vi "Begin.vi"(11 "Image Size":T1=enum."160x120") -> (0 "error out":errorcluster)   [LabVIEW 2013]
doc: "Called before other user functions, this VI is expected to open initial I/O refnums, load in file data, and do all program initialization. Notice that the <B>error out</B> terminal is simply used for data flow. Wiring it to other structures or subVIs ensures that this VI runs first."
uses:
  <vilib>/Rock Robotics/WPI/Camera/WPI_CameraImageSize.ctl
  <vilib>/Rock Robotics/WPI/Camera/WPI_CameraWhite Balance Values.ctl
  <vilib>/Rock Robotics/WPI/Camera/WPI_CameraExposure Values.ctl
  <vilib>/Rock Robotics/WPI/Camera/WPI_CameraFrameRate.ctl
  <vilib>/Rock Robotics/WPI/DriverStation/WPI_DriverStationRobotMode2.ctl
  <vilib>/Rock Robotics/SystemInterfaces/DIO/FPGA_DIOPWMChannel.ctl
  <vilib>/Rock Robotics/WPI/SafetyOutput/WPI_SafetyOutputConfigMenu.ctl
  <vilib>/Rock Robotics/WPI/Joystick/WPI_JoystickDeviceEnum.ctl
  TankDriveEnum.ctl
  Robot Global Data.vi
  <vilib>/Rock Robotics/WPI/RobotDrive/WPI_RobotDriveOpen2MotorWithTalon.vi
  <vilib>/Rock Robotics/WPI/Counter/WPI_CounterDigitalInputToDigitalSource.vi
  <vilib>/Rock Robotics/SystemInterfaces/Typedef/FPGA_TypedefDigitalModule.ctl
  <vilib>/Rock Robotics/SystemInterfaces/DIO/FPGA_DIOChannel.ctl
  <vilib>/Rock Robotics/WPI/Encoder/WPI_EncoderType.ctl
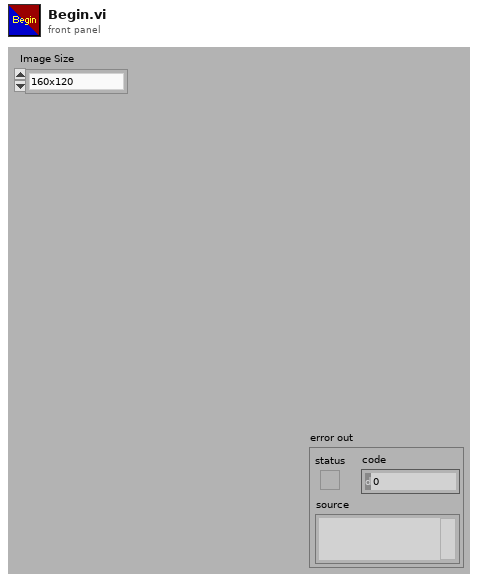
[diagram p1: front panel]
types:
  T1 = typedef "WPI_CameraImageSize.ctl" = enum16{"640x480", "320x240", "160x120"}
  T2 = typedef "TankDriveEnum.ctl" = enum16{"Init", "SetValue", "Disable", "Linear Drive"}
  T3 = typedef "WPI_JoystickDeviceEnum.ctl" = enum16{"USB 1", "USB 2", "USB 3", "USB 4", "Kinect 1", "Kinect 2"}
  T4 = typedef "WPI_SafetyOutputConfigMenu.ctl" = enum16{"Enable", "Disable"}
  T5 = typedef "FPGA_DIOPWMChannel.ctl" = enum8{"PWM 1", "PWM 2", "PWM 3", "PWM 4", "PWM 5", "PWM 6", "PWM 7", "PWM 8", "PWM 9", "PWM 10", "Invalid"}
  T6 = typedef "WPI_DriverStationRobotMode2.ctl" = enum16{"Autonomous Disabled", "Autonomous Enabled", "Teleop Disabled", "Teleop Enabled", "Timeout", "Finish", "Test Disabled", "Test Enabled"}
  T7 = typedef "WPI_CameraFrameRate.ctl" = u32
  T8 = typedef "WPI_CameraExposure Values.ctl" = enum16{"Auto", "Flicker-free 50 Hz", "Flicker-free 60 Hz", "Hold current"}
  T9 = typedef "WPI_CameraWhite Balance Values.ctl" = enum16{"Auto", "Fixed indoor", "Fixed outdoor 1", "Fixed outdoor 2", "Fixed fluorescent 1", "Fixed fluorescent 2", "Hold current"}
  T10 = typedef "WPI_CameraDevRef.ctl" = cluster{"Camera Address":string, "CameraStatus":errorcluster, "Acquire Image Notifier":refnum<notifier>}
  T11 = typedef "WPI_JoystickDevRef.ctl" = cluster{"Device":T3}
  T12 = typedef "FPGA_DIOChannel.ctl" = enum8{"DIO 1", "DIO 2", "DIO 3", "DIO 4", "DIO 5", "DIO 6", "DIO 7", "DIO 8", "DIO 9", "DIO 10", "DIO 11", "DIO 12", "DIO 13", "DIO 14", "Invalid"}
  T13 = typedef "FPGA_TypedefDigitalModule.ctl" = enum16{"Digital Module 1", "Digital Module 2"}
  T14 = typedef "WPI_EncoderType.ctl" = enum16{"1x", "2x", "4x"}
  T15 = typedef "WPI_DigitalInputDevRef.ctl" = cluster{"DevStatus":errorcluster, "DIO Channel":T12, "Digital Module":T13}
  T16 = typedef "FPGA_CounterEncoderSourceConvertionLVSourceType.ctl" = cluster{"DevStatus":errorcluster, "AnalogTriggerMode?":bool, "DigitalMode":cluster{"Digital Module":T13, "DIO Channel":T17}, "AnalogTriggerMode":cluster{"AnalogTriggerIndex":T18, "OutputType":T19}}
  T17 = typedef "FPGA_DIODigitalSourceChannel.ctl" = enum8{"DIO 1", "DIO 2", "DIO 3", "DIO 4", "DIO 5", "DIO 6", "DIO 7", "DIO 8", "DIO 9", "DIO 10", "DIO 11", "DIO 12", "DIO 13", "DIO 14", "Disabled"}
  T18 = typedef "FPGA_AnalogTriggerIndex.ctl" = enum8{"Trig 0", "Trig 1", "Trig 2", "Trig 3", "Trig 4", "Trig 5", "Trig 6", "Trig 7", "Invalid"}
  T19 = typedef "FPGA_AnalogTriggerOutType.ctl" = enum16{"InWindow", "TriggerState", "Rising", "Falling"}
  T20 = typedef "WPI_EncoderDevRef.ctl" = cluster{"DevStatus":errorcluster, "EncoderIndex":T21, "CounterIndex":T22, "DistancePerCount":dbl, "Decoding Type":T14}
  T21 = typedef "FPGA_EncoderIdx.ctl" = enum8{"Enc 0", "Enc 1", "Enc 2", "Enc 3", "Invalid"}
  T22 = typedef "FPGA_CounterCtrSystemIndex.ctl" = enum8{"Ctr 0", "Ctr 1", "Ctr 2", "Ctr 3", "Ctr 4", "Ctr 5", "Ctr 6", "Ctr 7", "Invalid"}
  T23 = typedef "WPI_RobotDriveDevRef.ctl" = cluster{"DevStatus":errorcluster, "Motors[]":T24[], "Square Inputs":bool, "Max Output":dbl, "Isochronous":bool}
  T24 = typedef "WPI_MotorControlDeviceRef.ctl" = cluster{"DeviceStatus":errorcluster, "Type":enum16{"PWM", "CAN"}, "PWM":cluster{"Digital Module":T13, "PWM Channel":T5, "DeadBand":T25}, "CAN":cluster{"Device Number":u8, "Control Mode":T26, "Semaphore":T27, "Max Vout":dbl}, "Invert":bool, "TransformRef":T28, "InvTransformRef":T28}
  T25 = typedef "WPI_PWMDeadband.ctl" = cluster{"Name":string, "maxPositivePwm":i32, "minPositivePwm":i32, "centerPwm":i32, "maxNegativePwm":i32, "minNegativePwm":i32, "angularRange":u16}
  T26 = typedef "WPI_CANJaguar_ControlMode.ctl" = enum8{"Percent VBus", "Current", "Speed", "Position", "Voltage"}
  T27 = typedef "Semaphore RefNum" = refnum<k1>
  T28 = typedef "WPI_PWMTransform_ConPane.ctl" = refnum<vi>
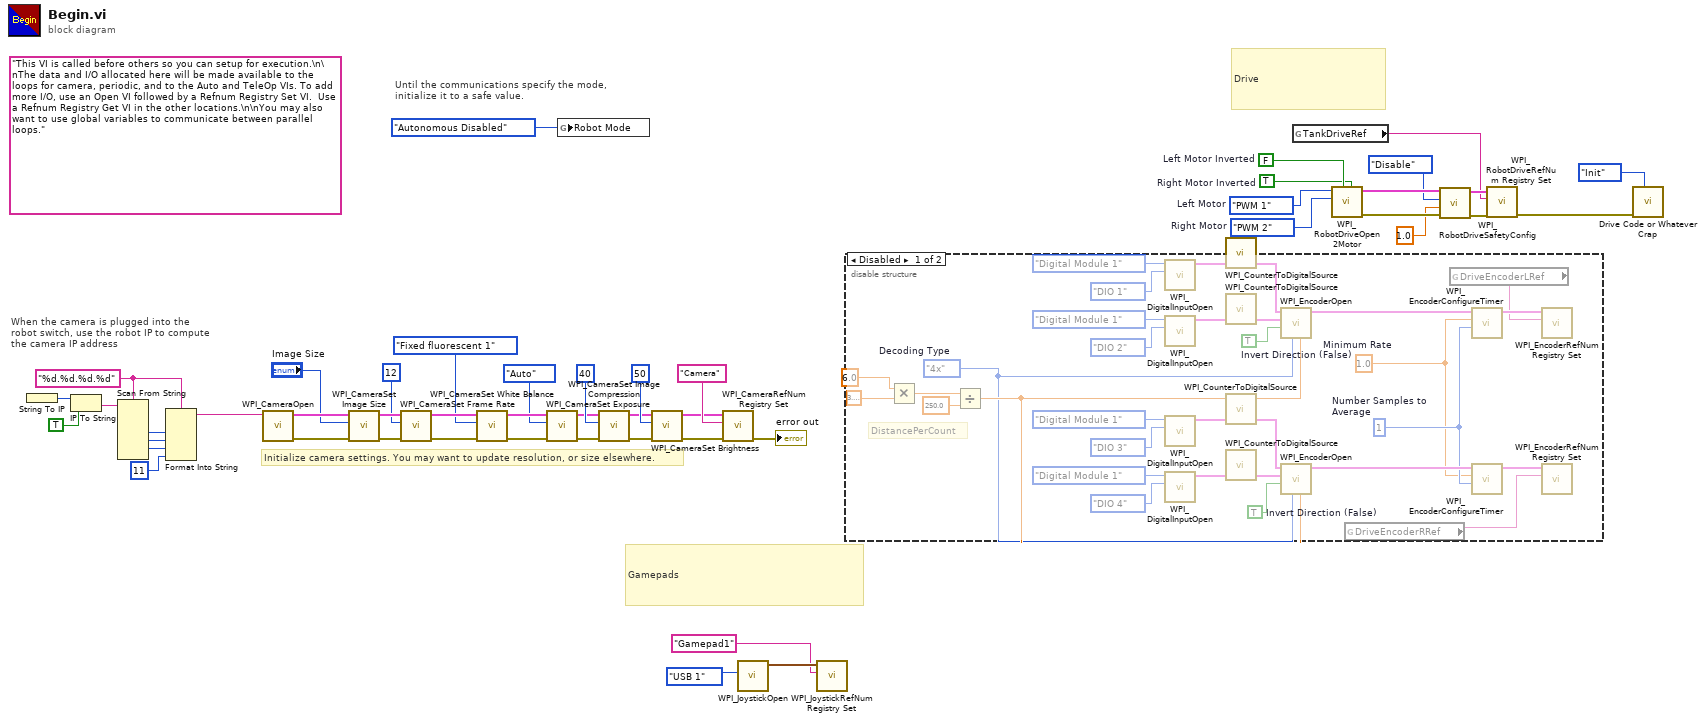
[diagram p0: block diagram]
diagram:
  w13 = FPGA_DIOPWMChannel."PWM 2"  # Right Motor
  w14 = FPGA_DIOPWMChannel."PWM 1"  # Left Motor
  w15 = TRUE  # Right Motor Inverted
  w16 = FALSE  # Left Motor Inverted
  w20 = "%d.%d.%d.%d" ("format string")
  (unwired) "This VI is called before others so you can setup for execution.\n\nThe data and I/O allocated here will be made available to the loops for camera, periodic, and to the Auto and TeleOp VIs. To add more I/O, use an Open VI followed by a Refnum Registry Set VI.  Use a Refnum Registry Get VI in the other locations.\n\nYou may also want to use global variables to communicate between parallel loops."
  # "Gamepads"
  # "Drive"
  # "Until the communications specify the mode,\ninitialize it to a safe value."
  # "When the camera is plugged into the\nrobot switch, use the robot IP to compute\nthe camera IP address"
  # "Initialize camera settings. You may want to update resolution, or size elsewhere."
  n1 = String To IP() -> (0:w27:u32)  [unwired: 1 in]
  n2 = IP To String(1:TRUE ("dot notation? (F)"), 2:w27) -> (0:w25:string)
  n3 = Scan From String(format string=w20, input string=w25) -> (output 1=w24:i32, output 2=w23:i32, output 3=w22:i32)  [unwired: 7 in, 3 out]
  n4 = Format Into String(format string=w20, w24, w23, w22, 11 ("Compression")) -> (resulting string=w18:string)  [unwired: 2 in, 1 out]
  n5 = call <vilib>:"WPI_CameraOpen.vi"("Camera Address"=w18) -> ("error out"=w39:errorcluster, "CameraDevRef"=w40:T10)  [unwired: 1 in, 8 out]
  n6 = call <vilib>:"WPI_CameraSet Image Size.vi"("error in (no error)"=w39, "Image Size"="Image Size", "CameraDevRef"=w40) -> ("error out"=w38:errorcluster, "CameraDevRef Out"=w41:T10)  [unwired: 7 out]
  n7 = call <vilib>:"WPI_CameraSet Frame Rate.vi"("error in (no error)"=w38, "Frame Rate (fps)"=T7 12, "CameraDevRef"=w41) -> ("error out"=w37:errorcluster, "CameraDevRef Out"=w43:T10)  [unwired: 7 out]
  n8 = call <vilib>:"WPI_CameraSet White Balance.vi"("error in (no error)"=w37, "White Balance"=WPI_CameraWhite_Balance_Values."Fixed fluorescent 1", "CameraDevRef"=w43) -> ("error out"=w36:errorcluster, "CameraDevRef Out"=w42:T10)  [unwired: 7 out]
  n9 = call <vilib>:"WPI_CameraSet Exposure.vi"("error in (no error)"=w36, "Exposure"=WPI_CameraExposure_Values."Auto", "CameraDevRef"=w42) -> ("error out"=w35:errorcluster, "CameraDevRef Out"=w45:T10)  [unwired: 7 out]
  n10 = global write "Robot Global Data.vi" "Robot Mode"(WPI_DriverStationRobotMode2."Autonomous Disabled" ("Robot Mode")) -> ()
  n11 = call <vilib>:"WPI_CameraSet Image Compression.vi"("error in (no error)"=w35, "Compression"=40, "CameraDevRef"=w45) -> ("error out"=w34:errorcluster, "CameraDevRef Out"=w44:T10)  [unwired: 7 out]
  n12 = call <vilib>:"WPI_CameraSet Brightness.vi"("error in (no error)"=w34, "Brightness"=50, "CameraDevRef"=w44) -> ("error out"=w32:errorcluster, "CameraDevRef Out"=w33:T10)  [unwired: 7 out]
  n13 = call <vilib>:"WPI_CameraRefNum Registry Set.vi"("error in (no error)"=w32, "refnum name"="Camera", "CameraDevRef"=w33) -> ("error out"=→"error out":errorcluster)  [unwired: 8 out]
  n14 = call <vilib>:"WPI_JoystickOpen.vi"("JoystickDevice"=WPI_JoystickDeviceEnum."USB 1") -> ("JoystickDevRef"=w5:T11)  [unwired: 10 in]
  n15 = call <vilib>:"WPI_JoystickRefNum Registry Set.vi"("refnum name"="Gamepad1", "JoystickDevRef"=w5) -> ()  [unwired: 8 in, 2 out]
  n16 = disable-structure shown="Disabled" {
    frame Disabled {
      w53 = TRUE  # Invert Direction (False)
      w54 = TRUE  # Invert Direction (False)
      w55 = WPI_EncoderType."4x"  # Decoding Type
      w52 = u8 1  # Number Samples to Average
      w51 = 1.0  # Minimum Rate
      # "DistancePerCount"
      n17 = Multiply(x=6.0, y=3.141592653589793) -> (x*y=w58:dbl)
      n18 = Divide(x=w58, y=250.0) -> (x/y=w56:dbl)
      n19 = call <vilib>:"WPI_DigitalInputOpen.vi"("DIO Channel"=FPGA_DIOChannel."DIO 1", "Digital Module (Module 1)"=FPGA_TypedefDigitalModule."Digital Module 1") -> ("DigitalInputDevRef"=w78:T15)  [unwired: 1 in, 8 out]
      n20 = call <vilib>:"WPI_DigitalInputOpen.vi"("DIO Channel"=FPGA_DIOChannel."DIO 2", "Digital Module (Module 1)"=FPGA_TypedefDigitalModule."Digital Module 1") -> ("DigitalInputDevRef"=w79:T15)  [unwired: 1 in, 8 out]
      n21 = call <vilib>:"WPI_DigitalInputOpen.vi"("DIO Channel"=FPGA_DIOChannel."DIO 3", "Digital Module (Module 1)"=FPGA_TypedefDigitalModule."Digital Module 1") -> ("DigitalInputDevRef"=w68:T15)  [unwired: 1 in, 8 out]
      n22 = call <vilib>:"WPI_DigitalInputOpen.vi"("DIO Channel"=FPGA_DIOChannel."DIO 4", "Digital Module (Module 1)"=FPGA_TypedefDigitalModule."Digital Module 1") -> ("DigitalInputDevRef"=w69:T15)  [unwired: 1 in, 8 out]
      n23 = call-poly <vilib>:"WPI_CounterToDigitalSource.vi"("DigitalInputDevRef"=w78) -> ("Digital Source"=w77:T16)  [unwired: 6 out]
      n24 = call-poly <vilib>:"WPI_CounterToDigitalSource.vi"("DigitalInputDevRef"=w79) -> ("Digital Source"=w80:T16)  [unwired: 6 out]
      n25 = call-poly <vilib>:"WPI_CounterToDigitalSource.vi"("DigitalInputDevRef"=w68) -> ("Digital Source"=w67:T16)  [unwired: 6 out]
      n26 = call-poly <vilib>:"WPI_CounterToDigitalSource.vi"("DigitalInputDevRef"=w69) -> ("Digital Source"=w70:T16)  [unwired: 6 out]
      n27 = call <vilib>:"WPI_EncoderOpen.vi"("DistancePerCount"=w56, "Decoding Type"=w55, "Invert Direction (False)"=w54, "BSource"=w80, "ASource"=w77) -> ("EncoderDevRef"=w74:T20)  [unwired: 3 in, 3 out]
      n28 = call <vilib>:"WPI_EncoderOpen.vi"("DistancePerCount"=w56, "Decoding Type"=w55, "Invert Direction (False)"=w53, "BSource"=w70, "ASource"=w67) -> ("EncoderDevRef"=w64:T20)  [unwired: 3 in, 3 out]
      n29 = global read "Robot Global Data.vi" "DriveEncoderRRef"() -> (w49:string)
      n30 = global read "Robot Global Data.vi" "DriveEncoderLRef"() -> (w50:string)
      n31 = call <vilib>:"WPI_EncoderConfigureTimer.vi"("Number Samples to Average"=w52, "Minimum Rate"=w51, "EncoderDevRef"=w74) -> ("EncoderDevRef"=w71:T20)  [unwired: 1 in, 7 out]
      n32 = call <vilib>:"WPI_EncoderConfigureTimer.vi"("Number Samples to Average"=w52, "Minimum Rate"=w51, "EncoderDevRef"=w64) -> ("EncoderDevRef"=w61:T20)  [unwired: 1 in, 7 out]
      n33 = call <vilib>:"WPI_EncoderRefNum Registry Set.vi"("refnum name"=w50, "EncoderDevRef"=w71) -> ()  [unwired: 8 in, 2 out]
      n34 = call <vilib>:"WPI_EncoderRefNum Registry Set.vi"("refnum name"=w49, "EncoderDevRef"=w61) -> ()  [unwired: 8 in, 2 out]
    }
    frame Enabled {
    }
  }
  n35 = global read "Robot Global Data.vi" "TankDriveRef"() -> (w6:string)
  n36 = call-poly <vilib>:"WPI_RobotDriveOpen2Motor.vi"("Right Motor Inverted"=w15, "Left Motor Inverted"=w16, "Right Motor"=w13, "Left Motor"=w14) -> ("error out"=w9:errorcluster, "RobotDriveDevRef"=w12:T23)  [unwired: 6 in]
  n37 = call <vilib>:"WPI_RobotDriveSafetyConfig.vi"("error in (no error)"=w9, "timeout (s)"=1.0, "mode"=WPI_SafetyOutputConfigMenu."Disable", "RobotDriveDevRef"=w12) -> ("error out"=w10:errorcluster, "RobotDriveDevRef"=w11:T23)  [unwired: 6 in]
  n38 = call <vilib>:"WPI_RobotDriveRefNum Registry Set.vi"("error in (no error)"=w10, "refnum name"=w6, "RobotDriveDevRef"=w11) -> ("error out"=w2:errorcluster)  [unwired: 7 in, 1 out]
  n39 = call "Drive Code or Whatever Crap.vi"("Enum"=TankDriveEnum."Init", "error in (no error)"=w2) -> ()  [unwired: 9 in, 1 out]
